vi "Get Channel Access Mode.vi"(8 "error in (no error)":errorcluster, 11 "Transfer Configuration in":refnum<class "Configuration.Transfer.lvclass">) -> (0 "error out":errorcluster, 2 "access":T1, 3 "Transfer Configuration out":refnum<class "Configuration.Transfer.lvclass">)   [LabVIEW 2016, in "Data Sharing Framework.Configuration.lvlib" / "Configuration.Transfer.lvclass"]
uses:
  Configuration.Transfer.lvclass
  <vilib>/NI Veristand/Custom Device API/Data Access Type.ctl
  Configuration.Transfer.lvclass/Configuration.Transfer.ctl
  <vilib>/NI VeriStand/Custom Device API/Custom Device API.lvlib
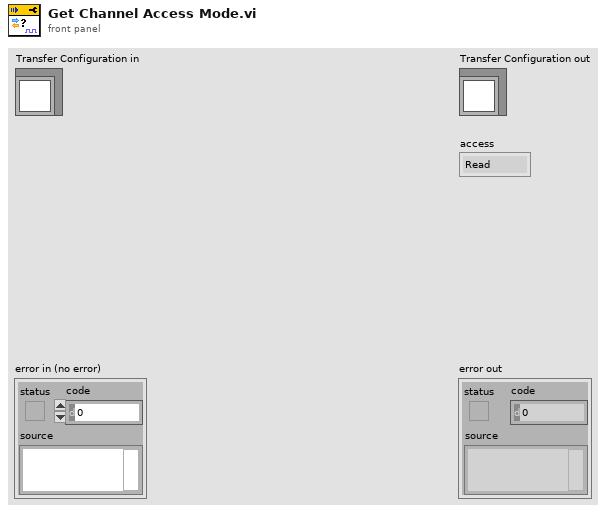
[diagram p1: front panel]
types:
  T1 = typedef "Custom Device API.lvlib/Data Access Type.ctl" = enum16{"Read", "Write"}
  T2 = typedef "Transfer Direction.ctl" = enum16{"Transmit", "Receive"}
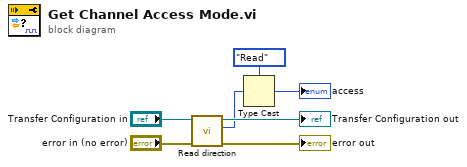
[diagram p0: block diagram]
diagram:
  n1 = call "Read direction.vi"("error in (no error)"="error in (no error)", "Configuration.Transfer in"="Transfer Configuration in") -> ("error out"=→"error out":errorcluster, "direction"=w3:T2, "Configuration.Transfer out"=→"Transfer Configuration out":refnum<class "Configuration.Transfer.lvclass">)  [unwired: 7 in]
  n2 = Type Cast(type=Data_Access_Type."Read" ("access"), x=w3) -> (*(type *) &x=→"access":T1)
